vi "Do.vi"(8 "error in (no error)":errorcluster, 10 "Actor in":refnum<class "Actor.lvclass">, 11 "Set Legend Msg in":refnum<class "Set Legend Msg.lvclass">) -> (0 "error out":errorcluster, 2 "Actor out":refnum<class "Actor.lvclass">)   [LabVIEW 2020, in "Task Viewer.lvlib" / "Set Legend Msg.lvclass"]
doc: "(<B>Filename</B>: Actor Framework.lvlib:Message.lvclass:Do.vi)\n\nDefines what a message does when it is received by an actor. Generally, a message instructs an actor to invoke one of its methods. By default, this method does nothing. A child class must override it to define behavior. Create a child class by using the Actor Framework Message Maker dialog box."
uses:
  Set Legend Msg.lvclass
  <vilib>/ActorFramework/Actor/Actor.lvclass
  Task Viewer/Task Viewer.lvclass
  C:/Program Files/National Instruments/LabVIEW 2020/vi.lib/ActorFramework/Actor/Actor.lvclass
  Set Legend Msg.lvclass/Set Legend Msg.ctl
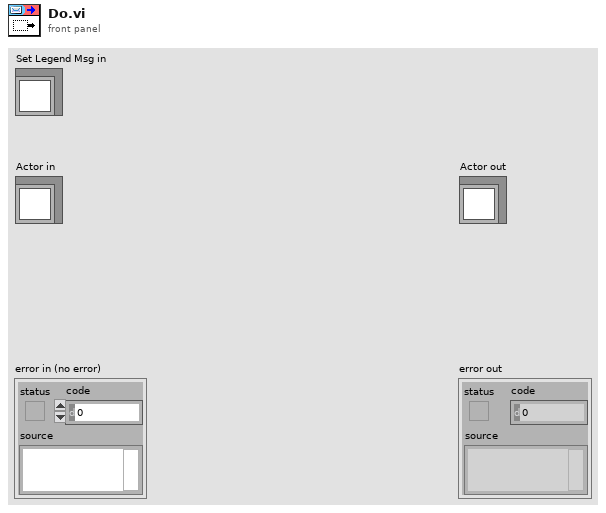
[diagram p1: front panel]
types:
  T1 = typedef "Collection Type df.ctl" = enum32{"Force Input", "Movement Input", "EMG only"}
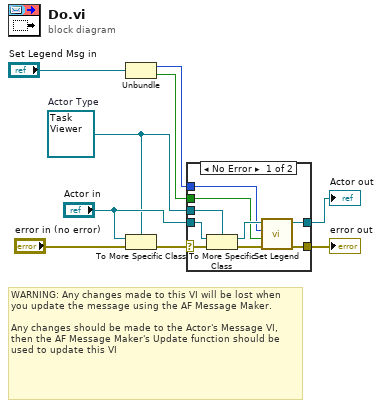
[diagram p0: block diagram]
diagram:
  w4 = refnum<class "Task Viewer.lvclass"> refnum  # Actor Type
  # "WARNING: Any changes made to this VI will be lost when you update the message using the AF Message Maker.\n\nAny changes should be made to the Actor's Message VI, then the AF Message Maker's Update function should be used to update this VI"
  n1 = Unbundle("Set Legend Msg in") -> (w3:T1, w2:bool)
  n2 = To More Specific Class(target class=w4, reference="Actor in", error in="error in (no error)") -> (error out=w8:errorcluster)  [unwired: 1 out]
  n3 = case shown="No Error" w8 {
    selector: w8 -> [w18 w20]
    tunnel: [w13 w20] -> w7
    tunnel: [w12 w19] -> w6
    tunnel: "Actor in" -> [w17 w19]
    tunnel: w4 -> [w16 _]
    tunnel: w3 -> [w11 _]
    tunnel: w2 -> [w10 _]
    frame No Error {
      n4 = To More Specific Class ("Actor Cast")(target class=w16, reference=w17, error in=w18) -> (specific class reference=w15:refnum<class "Task Viewer.lvclass">, error out=w14:errorcluster)
      n5 = call "Set Legend.vi"("error in (no error)"=w14, "EMG?"=w10, "Collection mode"=w11, "Task Viewer in"=w15) -> ("error out"=w13:errorcluster, "Task Viewer out"=w12:refnum<class "Task Viewer.lvclass">)  [unwired: 6 in]
    }
    frame Error {
    }
  }
  "error out" <- w7
  "Actor out" <- w6
